vi "CoG.vi"(0 "fullfilment consequence":dbl[](array[numeric])=[0.0, 1.0, 0.0] step=0.01 format="%.2f", 1 "consequence":T1(array[cluster])=[{"ling.var."="out", "x-min"=-1.0, "x-max"=1.0, "setarray"=[{"linguistic term"="NEo", "color"=16711680, "points"=[-1.0, -1.0, -1.0, 0.0]}, {"linguistic term"="ZEo", "color"=255, "points"=[-1.0, 0.0, 0.0, 1.0]}, {"linguistic term"="POo", "color"=26214, "points"=[0.0, 1.0, 1.0, 1.0]}]}] {"x-min" format="%.2f"; "x-max" format="%.2f"; "setarray"."points" min=-1.0 max=1.0 step=0.10000000149011612 format="%.2f"}, 2 "active consequence":i32[](array[numeric])=[0, 1, 2], 3 "output when no consequence (0)":u16(ring) items=["last result", "Default"], 4 "output default (0,00)":dbl step=0.009999999776482582 format="%.2f") -> (5 "controller output":dbl format="%.2f", 6 "output assessment":string)   [LabVIEW 2017, in "NI_fuzzy logic.lvlib"]
doc: "Defuzzify (center of gravity, 2. approximation) \nThe CoG-Method calculates the prezise outputvalue with the gravitypoint and the area of each fired consequenceterm.\nOutput : Analog value for controlling\nInputs : -consequencearray\n - fullfillment of each term ...\n - active consequenceterms\n - output when no consequence term is firering\n (0: last value , 1: Defaultvalue)"
uses:
  <vilib>/addons/control/fuzzy/NI_fuzzy logic.lvlib
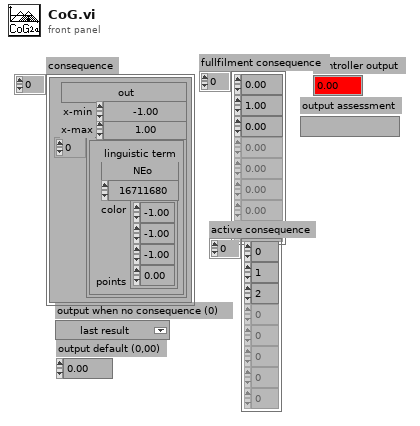
[diagram p1: front panel]
types:
  T1 = cluster{"ling.var.":string, "x-min":dbl, "x-max":dbl, "setarray":cluster{"linguistic term":string, "color":u32, "points":dbl[]}[]}[]
  T2 = cluster{"ling.var.":string, "x-min":dbl, "x-max":dbl, "setarray":cluster{"linguistic term":string, "color":u32, "points":dbl[]}[]}
  T3 = cluster{"linguistic term":string, "color":u32, "points":dbl[]}[]
  T4 = cluster{"linguistic term":string, "color":u32, "points":dbl[]}
  T5 = cluster{"points[0]":dbl, "points[1]":dbl, "points[2]":dbl, "points[3]":dbl}
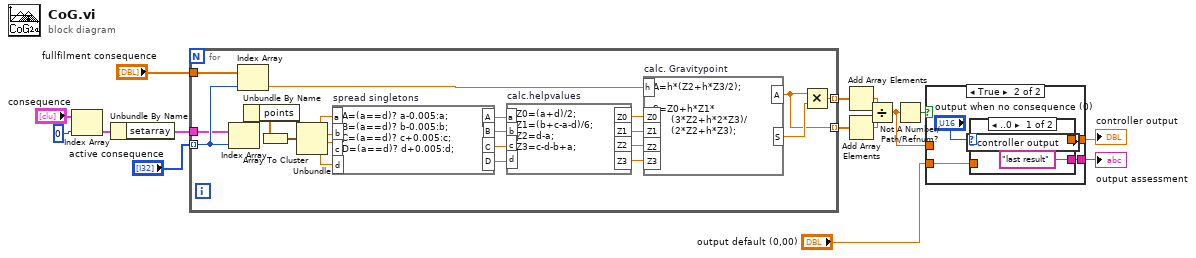
[diagram p0: block diagram]
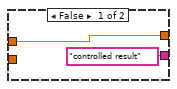
[diagram p2: hidden frame]
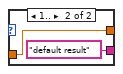
[diagram p3: hidden frame]
diagram:
  n1 = Index Array(array="consequence", index=0) -> (element=w7:T2)
  n2 = Unbundle By Name(w7) -> ("setarray"=w6:T3)
  n3 = for {
    tunnel: "fullfilment consequence" -> [w37]
    tunnel: "active consequence" -> [w36] mode=indexing
    tunnel: [w17] -> w10 mode=indexing
    tunnel: [w34] -> w9 mode=indexing
    tunnel: w6 -> [w33]
    n4 = Index Array(array=w33, index=w36) -> (element=w32:T4)
    n5 = Index Array(array=w37, index=w36) -> (element=w16:dbl)
    n6 = Unbundle By Name(w32) -> ("points"=w31:dbl[])
    n7 = Array To Cluster(array=w31) -> (cluster=w35:T5)
    n8 = Unbundle(w35) -> ("points[0]"=w27:dbl, "points[1]"=w24:dbl, "points[2]"=w25:dbl, "points[3]"=w26:dbl)
    n9 = formula code="A=(a==d)? a-0.005:a;\nB=(a==d)? b-0.005:b;\nC=(a==d)? c+0.005:c; \nD=(a==d)? d+0.005:d;" "spread singletons"("a"=w27, "b"=w24, "c"=w25, "d"=w26) -> ("A"=w30:dbl, "B"=w23:dbl, "C"=w29:dbl, "D"=w28:dbl)
    n10 = formula code="Z0=(a+d)/2;\nZ1=(b+c-a-d)/6;\nZ2=d-a;\nZ3=c-d-b+a;" "calc.helpvalues"("a"=w30, "b"=w23, "c"=w29, "d"=w28) -> ("Z0"=w22:dbl, "Z1"=w21:dbl, "Z2"=w20:dbl, "Z3"=w19:dbl)
    n11 = formula code="A=h*(Z2+h*Z3/2);\n\nS=Z0+h*Z1*\n      (3*Z2+h*2*Z3)/\n      (2*Z2+h*Z3);" "calc. Gravitypoint"("Z0"=w22, "Z1"=w21, "Z2"=w20, "Z3"=w19, "h"=w16) -> ("A"=w17:dbl, "S"=w18:dbl)
    n12 = Multiply(x=w17, y=w18) -> (x*y=w34:dbl)
  }
  n13 = Add Array Elements(numeric array=w9) -> (sum=w12:dbl)
  n14 = Add Array Elements(numeric array=w10) -> (sum=w11:dbl)
  n15 = Divide(x=w12, y=w11) -> (x/y=w5:dbl)
  n16 = Not A Number/Path/Refnum?(number/path/refnum=w5) -> (NaN/Path/Refnum?=w1:bool)
  n17 = case shown="True" w1 {
    tunnel: w5 -> [w39 _]
    tunnel: [w39 w43] -> w3
    tunnel: "output default (0,00)" -> [_ w42]
    tunnel: ["controlled result" w41] -> w2
    frame False {
    }
    frame True {
      n18 = case shown="..0" "output when no consequence (0)" {
        tunnel: [w45 w47] -> w43
        tunnel: w42 -> [_ w47]
        tunnel: ["last result" "default result"] -> w41
        frame ..0 {
          n19 = local read "controller output"() -> (w45:dbl)
        }
        frame 1.. {
        }
      }
    }
  }
  "controller output" <- w3
  "output assessment" <- w2
